vi "ReadAll.vi"(8 "error in (no error)":errorcluster, 11 "NetworkStreamReader in":refnum<class "NetworkStreamReader.lvclass">) -> (0 "error out":errorcluster, 1 "New element?":bool, 2 "elements":variant[](array[variant]), 3 "NetworkStreamReader out":refnum<class "NetworkStreamReader.lvclass">, 4 "Latest time stamp":timestamp)   [LabVIEW 2013, in "NetworkStreamReader.lvclass"]
uses:
  NetworkStreamReader.lvclass
  NetworkStreamReader.lvclass/NetworkStreamReader.ctl
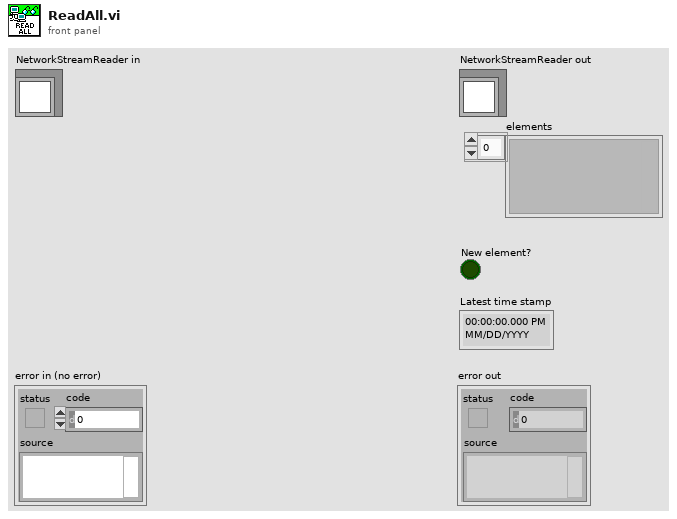
[diagram p1: front panel]
types:
  T1 = typedef "TimeStampedMessage.ctl" = cluster{"Data":variant, "Time Stamp":timestamp}
  T2 = typedef "TimeStampedMessageQueue.ctl" = refnum<queue>
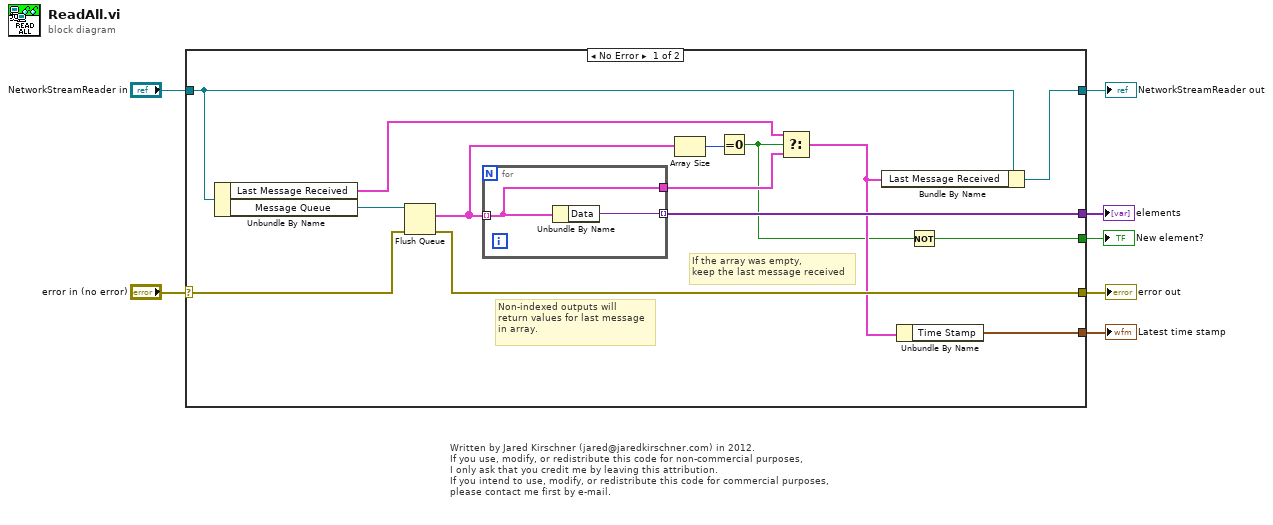
[diagram p0: block diagram]
diagram:
  # "Written by Jared Kirschner (jared@jaredkirschner.com) in 2012.\nIf you use, modify, or redistribute this code for non-commercial purposes,\nI only ask that you credit me by leaving this attribution.\nIf you intend to use, modify, or redistribute this code for commercial purposes,\nplease contact me first by e-mail."
  n1 = case shown="No Error" "error in (no error)" {
    selector: "error in (no error)" -> [w19 w25]
    tunnel: [w17 w25] -> w6
    tunnel: [w20 w24] -> w5
    tunnel: "NetworkStreamReader in" -> [w21 w24]
    tunnel: [w18 _] -> w2
    tunnel: [w8 _] -> w3
    tunnel: [w9 _] -> w1
    frame No Error {
      # "If the array was empty,\nkeep the last message received"
      # "Non-indexed outputs will\nreturn values for last message\nin array."
      n2 = Unbundle By Name(w21) -> ("Last Message Received"=w13:T1, "Message Queue"=w14:T2)
      n3 = Flush Queue(queue=w14, error in (no error)=w19) -> (remaining elements=w16:T1[], error out=w17:errorcluster)  [unwired: 1 out]
      n4 = for {
        tunnel: w16 -> [w22] mode=indexing
        tunnel: [w23] -> w18 mode=indexing
        tunnel: [w22] -> w12
        n5 = Unbundle By Name(w22) -> ("Data"=w23:variant)
      }
      n6 = Array Size(array=w16) -> (size(s)=w15:i32)
      n7 = Equal To 0?(x=w15) -> (x = 0?=w10:bool)
      n8 = Select(t=w13, s=w10, f=w12) -> (s? t:f=w11:T1)
      n9 = Bundle By Name(cluster=w21, "Last Message Received"=w11) -> (w20:refnum<class "NetworkStreamReader.lvclass">)
      n10 = Unbundle By Name(w11) -> ("Time Stamp"=w8:timestamp)
      n11 = Not(x=w10) -> (.not. x?=w9:bool)
    }
    frame Error {
    }
  }
  "error out" <- w6
  "NetworkStreamReader out" <- w5
  "Latest time stamp" <- w3
  "elements" <- w2
  "New element?" <- w1
